vi "Add Email Main Content.vi"(4 "Body:":string="asda", 6 "Subject:":string="asd", 8 "error in (no error)":errorcluster, 9 "To: (email@site.com)":string="923371272@qq.com", 10 "From: (email@site.com)":string="qianlingf@gmail.com", 11 "StmpEmail in":refnum<class "StmpEmail.lvclass">) -> (0 "error out":errorcluster, 3 "StmpEmail out":refnum<class "StmpEmail.lvclass">)   [LabVIEW 2015, in "StmpEmail.lvclass"]
uses:
  StmpEmail.lvclass
  StmpEmail.lvclass/StmpEmail.ctl
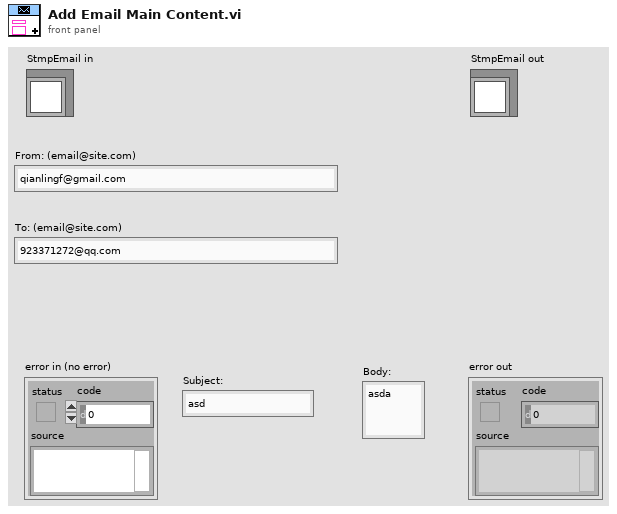
[diagram p1: front panel]
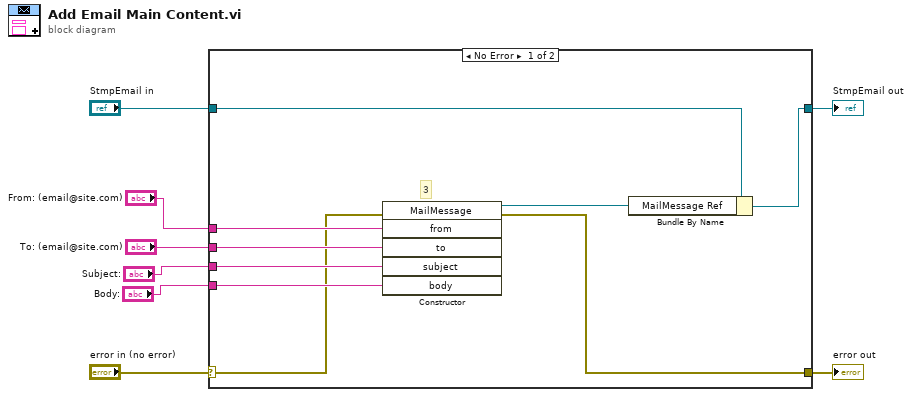
[diagram p0: block diagram]
diagram:
  n1 = case shown="No Error" "error in (no error)" {
    selector: "error in (no error)" -> [w13 w19]
    tunnel: [w12 w19] -> w7
    tunnel: [w9 w18] -> w5
    tunnel: "StmpEmail in" -> [w11 w18]
    tunnel: "From: (email@site.com)" -> [w17 _]
    tunnel: "To: (email@site.com)" -> [w16 _]
    tunnel: "Subject:" -> [w15 _]
    tunnel: "Body:" -> [w14 _]
    frame No Error {
      # "3"
      n2 = constructor class="MailMessage"(error in=w13, "from"=w17, "to"=w16, "subject"=w15, "body"=w14) -> (reference out=w10:refnum<k24>, error out=w12:errorcluster)  [unwired: 2 in, 5 out]
      n3 = Bundle By Name(cluster=w11, "MailMessage Ref"=w10) -> (w9:refnum<class "StmpEmail.lvclass">)
    }
    frame Error {
    }
  }
  "error out" <- w7
  "StmpEmail out" <- w5
